vi "initialization.vi"(8 "error in (no error)":errorcluster, 11 "ConnectionString":string) -> (0 "error out":errorcluster, 3 "ADODB._Connection Out":refnum<k7>)   [LabVIEW 2016, in "database.lvlib"]
uses:
  database.lvlib
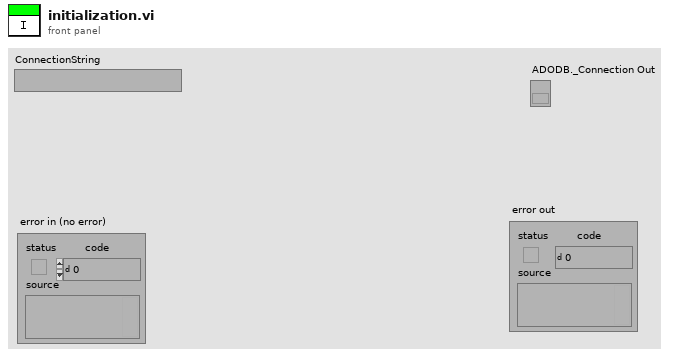
[diagram p1: front panel]
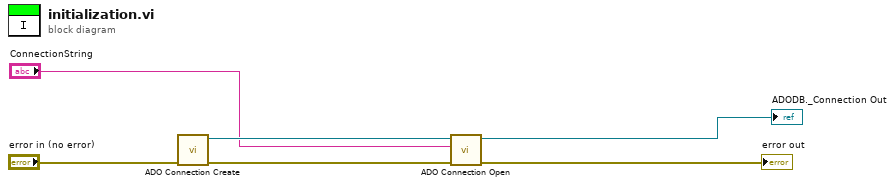
[diagram p0: block diagram]
diagram:
  n1 = call <userlib>:"ADO Connection Create.vi"("error in (no error)"="error in (no error)") -> ("error out"=w5:errorcluster, "ADODB._Connection Out"=w6:refnum<k7>)  [unwired: 9 in]
  n2 = call <userlib>:"ADO Connection Open.vi"("error in (no error)"=w5, "ConnectionString"="ConnectionString", "ADODB._Connection In"=w6) -> ("error out"=→"error out":errorcluster, "ADODB._Connection Out"=→"ADODB._Connection Out":refnum<k7>)  [unwired: 7 in]
